vi "Timeout.vi"(8 "error in (no error)":errorcluster, 11 "cRIO-CO2 in":refnum<class "cRIO-CO2.lvclass">) -> (0 "error out":errorcluster, 3 "cRIO-CO2 out":refnum<class "cRIO-CO2.lvclass">)   [LabVIEW 2015, in "cRIO-Carbondioxide.lvlib" / "cRIO-CO2.lvlib" / "cRIO-CO2.lvclass"]
uses:
  cRIO-CO2.lvclass
  <vilib>/nisyscfg/nisyscfg.lvlib
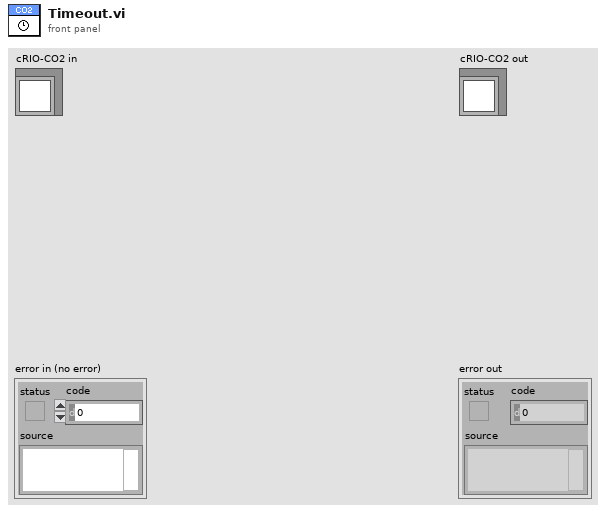
[diagram p1: front panel]
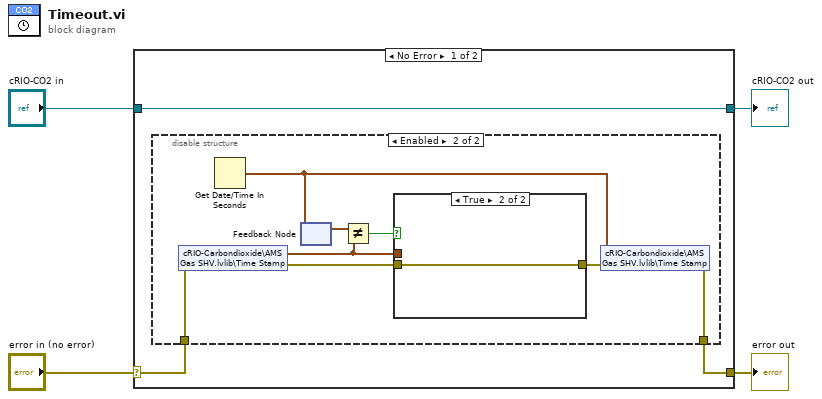
[diagram p0: block diagram]
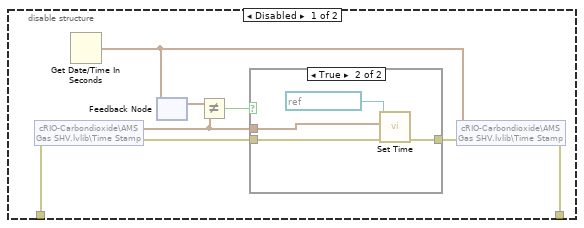
[diagram p2: hidden frame]
diagram:
  n1 = case shown="No Error" "error in (no error)" {
    selector: "error in (no error)" -> [w6 w32]
    tunnel: [w5 w32] -> w3
    tunnel: [w7 w31] -> w1
    tunnel: "cRIO-CO2 in" -> [w7 w31]
    frame No Error {
      n2 = disable-structure shown="Enabled" {
        disable-tunnel: w6 -> [w13 w26]
        disable-tunnel: [w9 w22] -> w5
        frame Disabled {
          n3 = shared-variable "cRIO-Carbondioxide\\AMS Gas SHV.lvlib\\Time Stamp"(error in=w13) -> (w11:timestamp, error out=w14:errorcluster)
          n4 = Get Date/Time In Seconds() -> (seconds since 1Jan1904=w8:timestamp)
          n5 = feedback #1() -> (w12:timestamp)  [unwired: 1 in]
          n6 = feedback-in #1(w8) -> ()
          n7 = Not Equal?(x=w12, y=w11) -> (x != y?=w15:bool)
          n8 = case shown="True" w15 {
            tunnel: w14 -> [w16 w20]
            tunnel: w11 -> [_ w19]
            tunnel: [w16 w18] -> w10
            frame False {
            }
            frame True {
              n9 = call <vilib>:"Set Time.vi"("error in (no error)"=w20, "Time"=w19, "Session in (localhost)"=refnum<k21> "localhost") -> ("error out"=w18:errorcluster)  [unwired: 5 in, 3 out]
            }
          }
          n10 = shared-variable "cRIO-Carbondioxide\\AMS Gas SHV.lvlib\\Time Stamp"(w8, error in=w10) -> (error out=w9:errorcluster)
        }
        frame Enabled {
          n11 = shared-variable "cRIO-Carbondioxide\\AMS Gas SHV.lvlib\\Time Stamp"(error in=w26) -> (w24:timestamp, error out=w27:errorcluster)
          n12 = Get Date/Time In Seconds() -> (seconds since 1Jan1904=w21:timestamp)
          n13 = feedback #2() -> (w25:timestamp)  [unwired: 1 in]
          n14 = feedback-in #2(w21) -> ()
          n15 = Not Equal?(x=w25, y=w24) -> (x != y?=w28:bool)
          n16 = case shown="True" w28 {
            tunnel: w27 -> [w29 w30]
            tunnel: w24 -> [_ _]
            tunnel: [w29 w30] -> w23
            frame False {
            }
            frame True {
            }
          }
          n17 = shared-variable "cRIO-Carbondioxide\\AMS Gas SHV.lvlib\\Time Stamp"(w21, error in=w23) -> (error out=w22:errorcluster)
        }
      }
    }
    frame Error {
    }
  }
  "error out" <- w3
  "cRIO-CO2 out" <- w1
